vi "Put Custom Fields.vi"(6 "Authentication Header":T1[](array[typedef]), 8 "error in (no error)":errorcluster, 9 "New Value":string, 10 "Custom Field GID":string, 11 "Task GID":string) -> (0 "error out":errorcluster, 2 "Response body":string)   [LabVIEW 2016]
uses:
  <vilib>/addons/_JKI.lib/REST Client/classes/REST Client/HTTP Header.ctl
  <vilib>/addons/_JKI.lib/REST Client/classes/REST Client/REST Client.lvclass
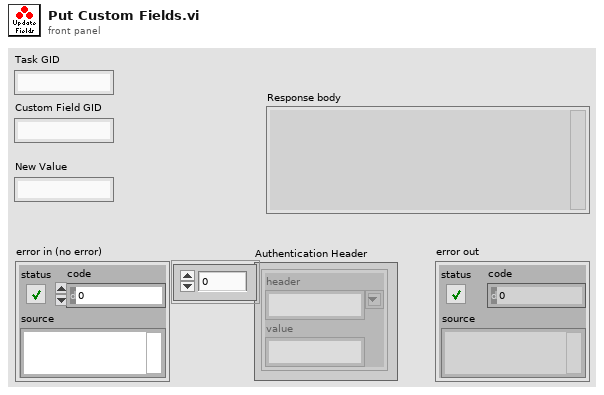
[diagram p1: front panel]
types:
  T1 = typedef "REST Client.lvlib/REST Client.lvclass/HTTP Header.ctl" = cluster{"header":string, "value":string}
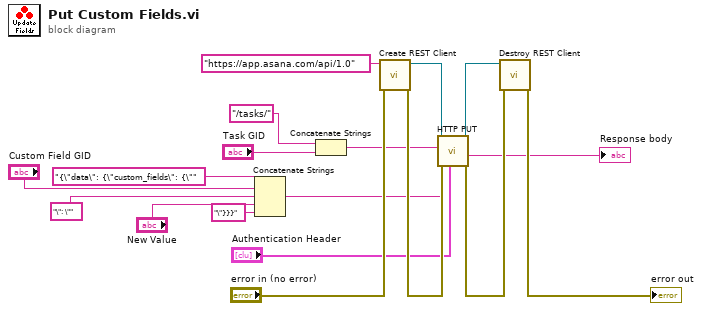
[diagram p0: block diagram]
diagram:
  n1 = Concatenate Strings("{\"data\": {\"custom_fields\": {\"", "Custom Field GID", "\": \"", "New Value", "\"}}}" ("string")) -> (w1:string)
  n2 = Concatenate Strings("/tasks/" ("string"), "Task GID") -> (w10:string)
  n3 = call <vilib>:"Create REST Client.vi"("error in (no error)"="error in (no error)", "Base URL"="https://app.asana.com/api/1.0") -> ("error out"=w15:errorcluster, "REST Client out"=w18:refnum<class "REST Client.lvclass">)  [unwired: 8 in]
  n4 = call-dynamic "HTTP PUT.vi"("request specific headers"="Authentication Header", "error in (no error)"=w15, "Request body"=w1, "Path"=w10, "REST Client in"=w18) -> ("error out"=w13:errorcluster, "Response body"=→"Response body":string, "REST Client out"=w17:refnum<class "REST Client.lvclass">)  [unwired: 1 in, 3 out]
  n5 = call-dynamic "Destroy REST Client.vi"("error in (no error)"=w13, "REST Client in"=w17) -> ("error out"=→"error out":errorcluster)  [unwired: 9 in]
